vi "Read WRITE SETUP errors.vi"(8 "error in (no error)":errorcluster, 11 "Simulated_CCD_Camera in":refnum<class "Sim_Ixon_Ultra.lvclass">) -> (0 "error out":errorcluster, 2 "WRITE SETUP errors":errorcluster[](array[cluster]), 3 "Simulated_CCD_Camera out":refnum<class "Sim_Ixon_Ultra.lvclass">)   [LabVIEW 2018, in "Sim_Ixon_Ultra.lvclass"]
uses:
  Sim_Ixon_Ultra.lvclass
  Sim_Ixon_Ultra.lvclass/Sim_Ixon_Ultra.ctl
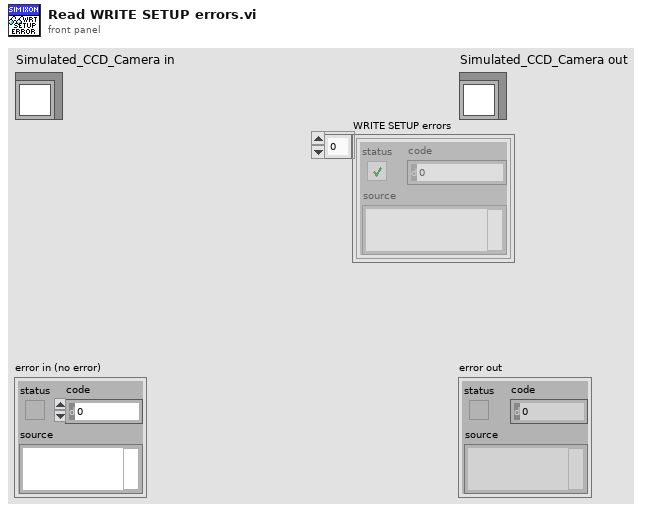
[diagram p1: front panel]
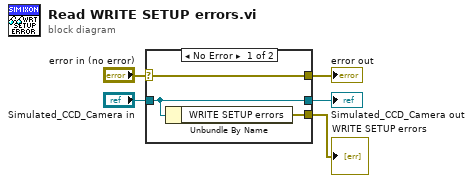
[diagram p0: block diagram]
diagram:
  n1 = case shown="No Error" "error in (no error)" {
    selector: "error in (no error)" -> [w7 w10]
    tunnel: "Simulated_CCD_Camera in" -> [w6 w9]
    tunnel: [w8 _] -> w1
    tunnel: [w7 w10] -> w3
    tunnel: [w6 w9] -> w2
    frame No Error {
      n2 = Unbundle By Name(w6) -> ("WRITE SETUP errors"=w8:errorcluster[])
    }
    frame Error {
    }
  }
  "error out" <- w3
  "Simulated_CCD_Camera out" <- w2
  "WRITE SETUP errors" <- w1
